vi "Pre Launch Init.vi"(11 "Remote Endpoint P3AT in":refnum<class "RemoteP3AT.lvclass"> caption="操作者输入") -> (0 "error out":errorcluster caption="错误输出", 3 "Remote Endpoint P3AT out":refnum<class "RemoteP3AT.lvclass"> caption="操作者输出")   [LabVIEW 2014, in "RemoteP3AT.lvlib" / "RemoteP3AT.lvclass"]
doc: "(<B>Filename</B>: Actor Framework.lvlib:Actor.lvclass:Pre Launch Init.vi)\n\nDefines behavior that occurs after the Launch Nested Actor method is invoked but before the actor's Actor Core method begins running.\n\nBy default, this method does nothing. A descendant class may override it to define behavior."
uses:
  RemoteP3AT.lvclass
  RemoteP3AT.lvclass/RemoteP3AT.ctl
  Wrapper_lib/zsActor/ActorWrapper.lvclass
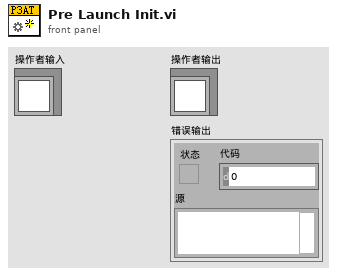
[diagram p1: front panel]
types:
  T1 = enum16{"OpenSlaveActor", "Idle", "StopSlaveActor"}
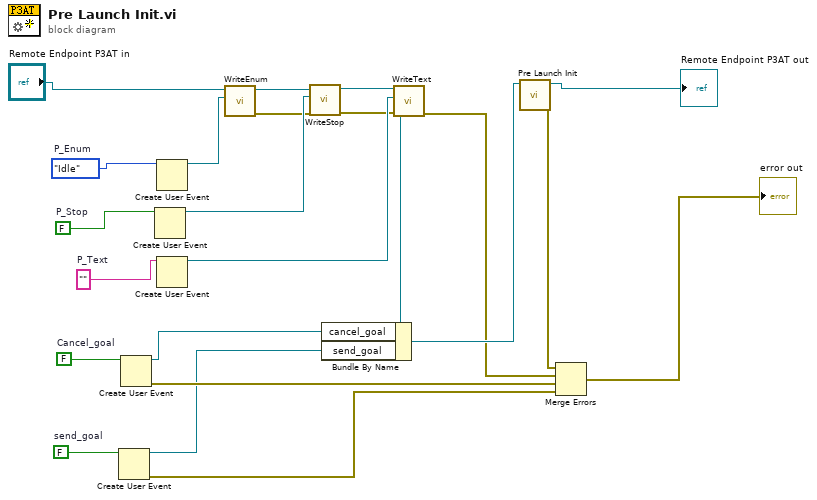
[diagram p0: block diagram]
diagram:
  w15 = ""  # P_Text
  w14 = FALSE  # P_Stop
  w13 = T1."Idle"  # P_Enum
  w20 = FALSE  # send_goal
  w22 = FALSE  # Cancel_goal
  n1 = Create User Event(user event datatype=w20) -> (user event=w1:refnum<user-event>, error out=w3:errorcluster)  [unwired: 1 in]
  n2 = Create User Event(user event datatype=w22) -> (user event=w2:refnum<user-event>, error out=w21:errorcluster)  [unwired: 1 in]
  n3 = Create User Event(user event datatype=w14) -> (user event=w11:refnum<user-event>)  [unwired: 1 in, 1 out]
  n4 = Create User Event(user event datatype=w13) -> (user event=w12:refnum<user-event>)  [unwired: 1 in, 1 out]
  n5 = Create User Event(user event datatype=w15) -> (user event=w10:refnum<user-event>)  [unwired: 1 in, 1 out]
  n6 = call-dynamic "WriteEnum.vi"("Enum"=w12, "zsActor输入"="Remote Endpoint P3AT in") -> ("error out"=w9:errorcluster, "zsActor输出"=w17:refnum<class "RemoteP3AT.lvclass">)  [unwired: 8 in]
  n7 = call-dynamic "WriteStop.vi"("error in (no error)"=w9, "Stop"=w11, "zsActor输入"=w17) -> ("error out"=w8:errorcluster, "zsActor输出"=w16:refnum<class "RemoteP3AT.lvclass">)  [unwired: 7 in]
  n8 = call-dynamic "WriteText.vi"("error in (no error)"=w8, "Text"=w10, "zsActor输入"=w16) -> ("error out"=w4:errorcluster, "zsActor输出"=w6:refnum<class "RemoteP3AT.lvclass">)  [unwired: 7 in]
  n9 = Bundle By Name(cluster=w6, "cancel_goal"=w2, "send_goal"=w1) -> (w18:refnum<class "RemoteP3AT.lvclass">)
  n10 = call-parent "Pre Launch Init.vi"("Actor in"=w18) -> ("error out"=w5:errorcluster, "Actor out"=→"Remote Endpoint P3AT out":refnum<class "RemoteP3AT.lvclass">)  [unwired: 9 in]
  n11 = Merge Errors(w5, w4, w21, w3) -> (→"error out":errorcluster)
